vi "Handle Command.vi"(8 "error in (no error)":errorcluster, 9 "Data":variant, 10 "Command":string, 11 "Example Instrument in":refnum<class "Instrument.FrameworkTemplate.lvclass">) -> (0 "error out":errorcluster, 1 "Processed Data":variant, 2 "Command":string, 3 "Example Instrument out":refnum<class "Instrument.FrameworkTemplate.lvclass">)   [LabVIEW 2019, in "Instrument.FrameworkTemplate.lvclass"]
uses:
  Instrument.FrameworkTemplate.lvclass
  Instrument.FrameworkTemplate.lvclass/Instrument.FrameworkTemplate.ctl
  9aec49fd-fe04-463a-be35-b7075f22e824.vi
  9aec49fd-fe04-463a-be35-b7075f22e824.vi/83bf8cbc-7b1a-467b-9a13-e15a8dc463e8.vi
  9aec49fd-fe04-463a-be35-b7075f22e824.vi/97ec0fa0-64ca-4eb9-b541-6a075c0a3782.vi
  <vilib>/Utility/Data Type/Get Type Information.vi
  <vilib>/JDP Science/JSONtext/JSON text to Variant.vi
  <vilib>/JDP Science/JSONtext/LVClass Serializer/JSONtext LVClass Serializer.lvclass
  <userlib>/LevyLab/Instrument Framework/Instrument Types/VSource/Instrument.VSource.lvclass
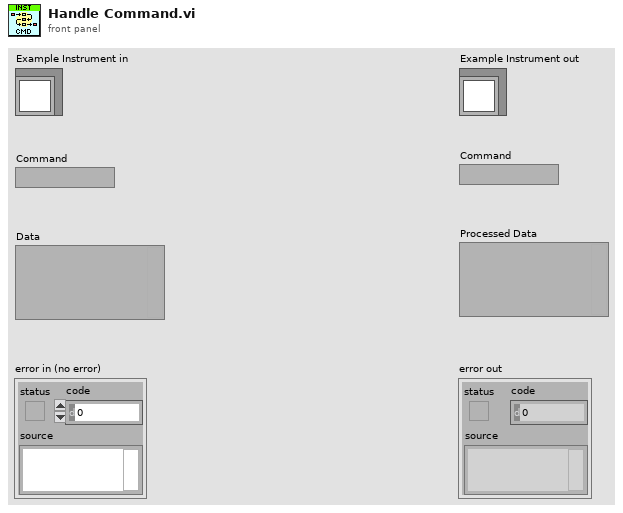
[diagram p1: front panel]
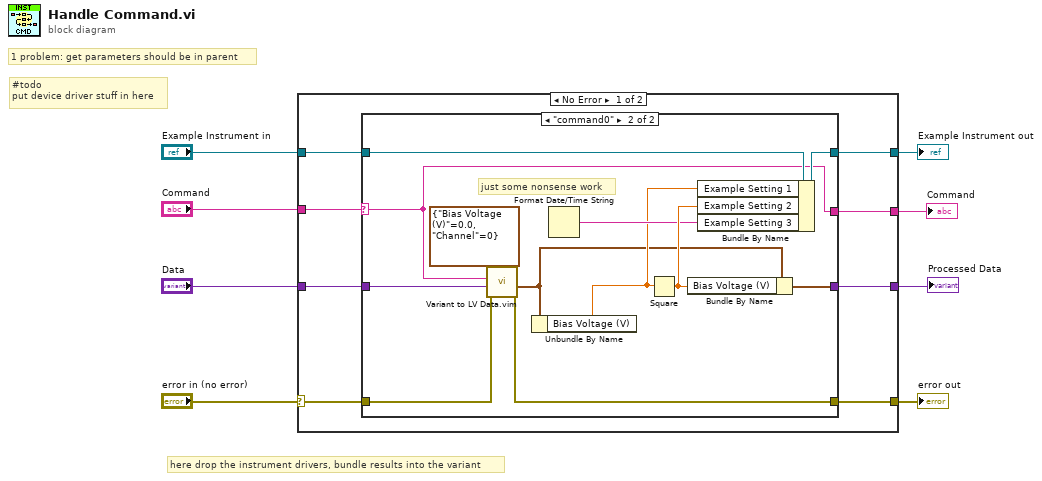
[diagram p0: block diagram]
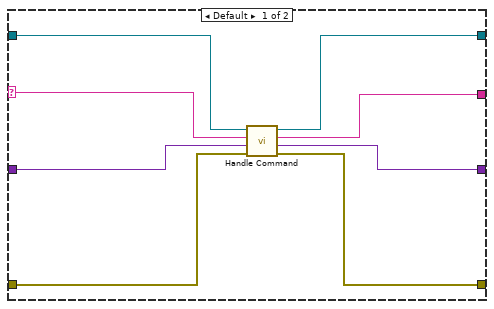
[diagram p2: hidden frame]
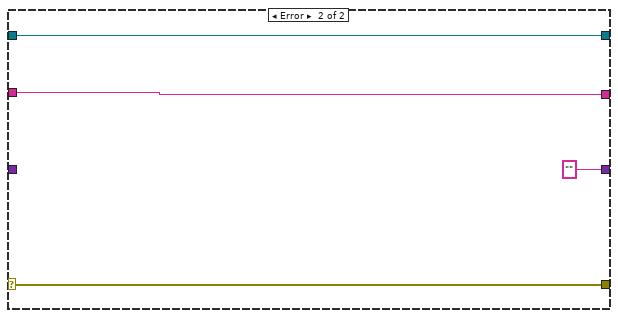
[diagram p3: hidden frame]
diagram:
  # "here drop the instrument drivers, bundle results into the variant"
  # "1 problem: get parameters should be in parent"
  # "#todo\nput device driver stuff in here"
  n1 = case shown="No Error" "error in (no error)" {
    selector: "error in (no error)" -> [w12 w40]
    tunnel: [w10 w40] -> w6
    tunnel: [w14 w39] -> w5
    tunnel: "Example Instrument in" -> [w15 w39]
    tunnel: "Command" -> [w16 w37]
    tunnel: [w13 "" ("String")] -> w3
    tunnel: "Data" -> [w11 _]
    tunnel: [w9 w37] -> w1
    frame No Error {
      n2 = case shown="\"command0\"" w16 {
        selector: w16 -> [w24 w28]
        tunnel: w15 -> [w21 w35]
        tunnel: [w18 w34] -> w14
        tunnel: [w20 w36] -> w13
        tunnel: w12 -> [w22 w31]
        tunnel: w11 -> [w23 w27]
        tunnel: [w19 w30] -> w10
        tunnel: [w17 w28] -> w9
        frame Default {
          n3 = call-parent "Handle Command.vi"("error in (no error)"=w22, "Data"=w23, "Command"=w24, "Instrument in"=w21) -> ("error out"=w19:errorcluster, "Processed Data"=w20:variant, "Command"=w17:string, "Instrument out"=w18:refnum<class "Instrument.FrameworkTemplate.lvclass">)  [unwired: 4 in]
        }
        frame "command0" {
          # "just some nonsense work"
          n4 = call "Variant to LV Data.vim"("type"=cluster{"Bias Voltage (V)":dbl, "Channel":i32} {"Bias Voltage (V)"=0.0, "Channel"=0} ("output cluster"), "error in (no error)"=w31, "JSON Data in"=w27, "Command"=w28) -> ("error out"=w30:errorcluster, "Data out"=w25:cluster{"Bias Voltage (V)":dbl, "Channel":i32})  [unwired: 4 in, 2 out]
          n5 = Unbundle By Name(w25) -> ("Bias Voltage (V)"=w26:dbl)
          n6 = Format Date/Time String() -> (date/time string=w32:string)  [unwired: 3 in]
          n7 = Square(x=w26) -> (x^2=w33:dbl)
          n8 = Bundle By Name(cluster=w25, "Bias Voltage (V)"=w33) -> (w36:cluster{"Bias Voltage (V)":dbl, "Channel":i32})
          n9 = Bundle By Name(cluster=w35, "Example Setting 1"=w26, "Example Setting 2"=w33, "Example Setting 3"=w32) -> (w34:refnum<class "Instrument.FrameworkTemplate.lvclass">)
        }
      }
    }
    frame Error {
    }
  }
  "error out" <- w6
  "Example Instrument out" <- w5
  "Command" <- w1
  "Processed Data" <- w3
